vi "First Step.vi"(8 "error in (no error)":errorcluster, 11 "Varian Magnet Scan.lvclass in":refnum<class "Varian Magnet Scan.lvclass">) -> (0 "error out":errorcluster, 2 "Current Position":dbl, 3 "Varian Magnet Scan.lvclass out":refnum<class "Varian Magnet Scan.lvclass">)   [LabVIEW 2009, in "Varian Magnet Scan.lvclass"]
doc: "Goto step #0 - the first step. If desired, the scanner may do this in a different way than usual (i.e. by preparing to move a long distance, or reset to home position.)"
uses:
  Varian Magnet Scan.lvclass
  Instruments/Varian Magnet/Varian Magnet.lvclass
  Scanner/Scanner.lvclass
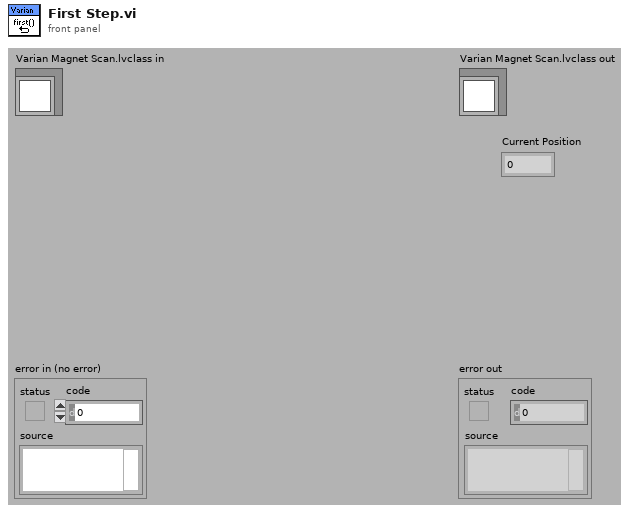
[diagram p1: front panel]
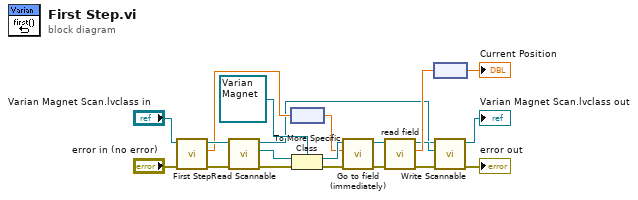
[diagram p0: block diagram]
diagram:
  n1 = call-parent "First Step.vi"("error in (no error)"="error in (no error)", "Scanner.lvclass in"="Varian Magnet Scan.lvclass in") -> ("error out"=w15:errorcluster, "Current Position"=w16:dbl, "Scanner.lvclass out"=w17:refnum<class "Varian Magnet Scan.lvclass">)  [unwired: 7 out]
  n2 = call-dynamic "Read Scannable.vi"("error in (no error)"=w15, "Scanner.lvclass in"=w17) -> ("error out"=w11:errorcluster, "Scannable.lvclass"=w14:refnum<class "Scannable.lvclass">, "Scanner.lvclass out"=w2:refnum<class "Varian Magnet Scan.lvclass">)  [unwired: 7 in]
  n3 = node(w16) -> (w9:dbl[unit])
  n4 = To More Specific Class(target class=refnum<class "Varian Magnet.lvclass"> refnum ("Varian Magnet.lvclass"), reference=w14, error in=w11) -> (specific class reference=w12:refnum<class "Varian Magnet.lvclass">, error out=w10:errorcluster)
  n5 = call "Go to field (immediately).vi"("error in"=w10, "Desired field (T)"=w9, "varian in"=w12) -> ("error out"=w8:errorcluster, "varian out"=w7:refnum<class "Varian Magnet.lvclass">)  [unwired: 7 in]
  n6 = call "read field.vi"("error in (no error)"=w8, "Varian Magnet.lvclass In"=w7) -> ("error out"=w3:errorcluster, "Field"=w6:dbl[unit], "Varian Magnet.lvclass Out"=w5:refnum<class "Varian Magnet.lvclass">)  [unwired: 7 in]
  n7 = node(w6) -> (→"Current Position":dbl)
  n8 = call-dynamic "Write Scannable.vi"("error in (no error)"=w3, "Scannable.lvclass"=w5, "Scanner.lvclass in"=w2) -> ("error out"=→"error out":errorcluster, "Scanner.lvclass out"=→"Varian Magnet Scan.lvclass out":refnum<class "Varian Magnet Scan.lvclass">)  [unwired: 7 in]
